vi "getSubArray3D.vi"(8 "error in (no error)":errorcluster, 9 "Index Array Cluster":T1, 11 "3D Array":dbl[][][](array[numeric])) -> (0 "error out":errorcluster, 3 "Sub-Array":dbl[][][](array[numeric]))   [LabVIEW 2016]
doc: "Get the sub-matrix from a 3D matrix."
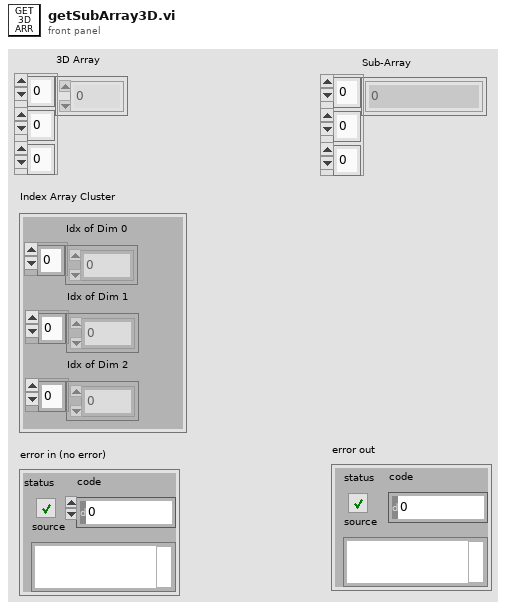
[diagram p1: front panel]
types:
  T1 = cluster{"Idx of Dim 0":i32[], "Idx of Dim 1":i32[], "Idx of Dim 2":i32[]}
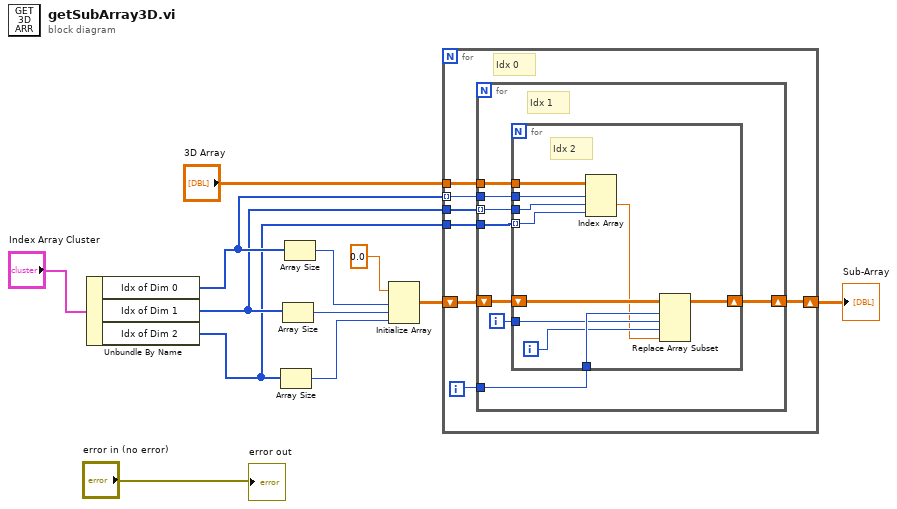
[diagram p0: block diagram]
diagram:
  n1 = Unbundle By Name("Index Array Cluster") -> ("Idx of Dim 0"=w4:i32[], "Idx of Dim 1"=w3:i32[], "Idx of Dim 2"=w2:i32[])
  n2 = Array Size(array=w2) -> (size(s)=w10:i32)
  n3 = Array Size(array=w3) -> (size(s)=w7:i32)
  n4 = Array Size(array=w4) -> (size(s)=w8:i32)
  n5 = Initialize Array(0.0 ("element"), w8, w7, w10) -> (w11:dbl[][][])
  n6 = for {
    tunnel: "3D Array" -> [w19]
    shift-right: [w17] -> w9
    shift-left: w11 -> [w18]
    tunnel: w4 -> [w16] mode=indexing
    tunnel: w3 -> [w15]
    tunnel: w2 -> [w14]
    i -> [w13]
    # "Idx 0"
    n7 = for {
      tunnel: w19 -> [w27]
      shift-right: [w25] -> w17
      shift-left: w18 -> [w26]
      tunnel: w16 -> [w24]
      tunnel: w15 -> [w23] mode=indexing
      tunnel: w14 -> [w22]
      tunnel: w13 -> [w21]
      i -> [w20]
      # "Idx 1"
      n8 = for {
        tunnel: w27 -> [w37]
        shift-right: [w31] -> w25
        shift-left: w26 -> [w33]
        tunnel: w24 -> [w36]
        tunnel: w23 -> [w35]
        tunnel: w22 -> [w34] mode=indexing
        tunnel: w21 -> [w32]
        tunnel: w20 -> [w30]
        i -> [w29]
        # "Idx 2"
        n9 = Index Array(array=w37, index (dim 0)=w36, index (dim 1)=w35, index (dim 2)=w34) -> (element=w28:dbl)
        n10 = Replace Array Subset(array=w33, new element=w28, index (dim 0)=w32, index (dim 1)=w30, index (dim 2)=w29) -> (w31:dbl[][][])
      }
    }
  }
  "Sub-Array" <- w9
  "error out" <- "error in (no error)"
